vi "Configure Dialog.vi"(8 "Error In":errorcluster, 11 "Actor Framework:Message in":refnum<class>) -> (0 "Error Out":errorcluster, 2 "Ok?":bool, 3 "Actor Framework:Message out":refnum<class>)   [LabVIEW 2015]
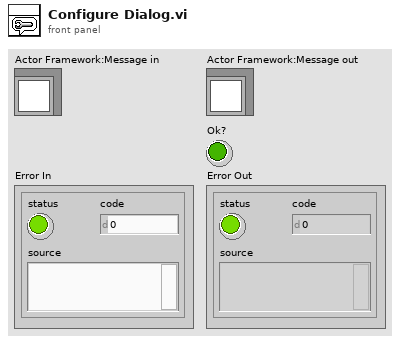
[diagram p1: front panel]
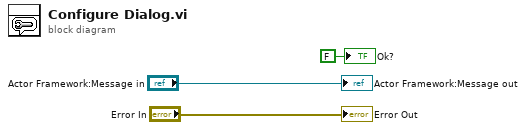
[diagram p0: block diagram]
diagram:
  "Error Out" <- "Error In"
  "Ok?" <- FALSE ("Ok?")
  "Actor Framework:Message out" <- "Actor Framework:Message in"
